vi "get_exe_home_path.vi"(8 "home_path":path) -> (2 "running in an executable?":bool, 3 "actual_home_path":path)   [LabVIEW 2012]
doc: "Given the pathname of a vi, returns the path contains the executable or the path of the vi.\nIf this is run from an executable \"built\" application, the path of directory containing the *.exe file is returned (regardless of which subvi path was input). If this is run from the development environment, the path returned is the simply the directory path that contains the vi."
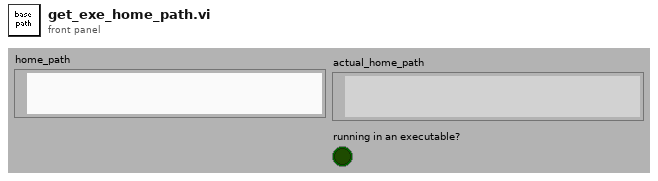
[diagram p1: front panel]
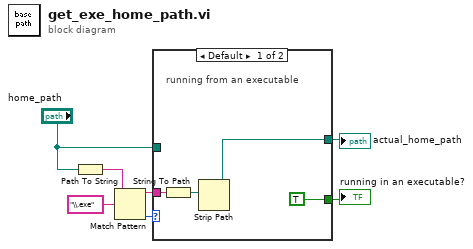
[diagram p0: block diagram]
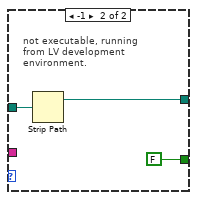
[diagram p2: hidden frame]
diagram:
  n1 = Path To String(path="home_path") -> (string=w7:string)
  n2 = Match Pattern(string=w7, regular expression="\\.exe") -> (before substring=w4:string, offset past match=w5:i32)  [unwired: 1 in, 2 out]
  n3 = case shown="Default" w5 {
    tunnel: "home_path" -> [_ w14]
    tunnel: [w8 w13] -> w1
    tunnel: w4 -> [w11 _]
    tunnel: [TRUE FALSE] -> w3
    frame Default {
      # "running from an executable"
      n4 = String To Path(string=w11) -> (path=w10:path)
      n5 = Strip Path(path=w10) -> (stripped path=w8:path)  [unwired: 1 out]
    }
    frame -1 {
      # "not executable, running\nfrom LV development\nenvironment."
      n6 = Strip Path(path=w14) -> (stripped path=w13:path)  [unwired: 1 out]
    }
  }
  "actual_home_path" <- w1
  "running in an executable?" <- w3
